vi "Obtain Channel DBL.vi"(8 "error in (no error)":errorcluster, 10 "Name":string, 11 "VolatusAPI in":refnum<class "VolatusAPI.lvclass">) -> (0 "error out":errorcluster, 2 "Channel DBL":refnum<class "Channel DBL.lvclass">, 3 "VolatusAPI out":refnum<class "VolatusAPI.lvclass">)   [LabVIEW 2020, in "Volatus.lvlib" / "VolatusAPI.lvclass"]
uses:
  VolatusAPI.lvclass
  VolatusAPI.lvclass/VolatusAPI.ctl
  lv-vecto/Vecto/Group DBL/Group DBL.lvclass
  C:/dev/lv20CE/relink/lv-vecto/Vecto/Group/Group.lvclass
  C:/dev/lv20CE/relink/lv-vecto/Vecto/Group DBL/Group DBL.lvclass
  lv-vecto/Vecto/Channel DBL/Channel DBL.lvclass
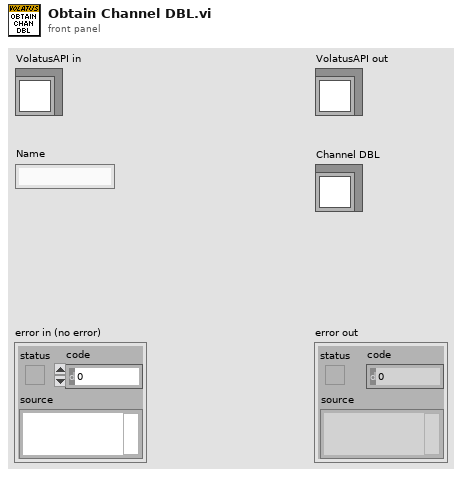
[diagram p1: front panel]
types:
  T1 = typedef "VectoConfig.lvlib/Channel Info.ctl" = cluster{"Name":string, "Group":string, "Owning Node":string, "Owning Task":string, "Resource":string}
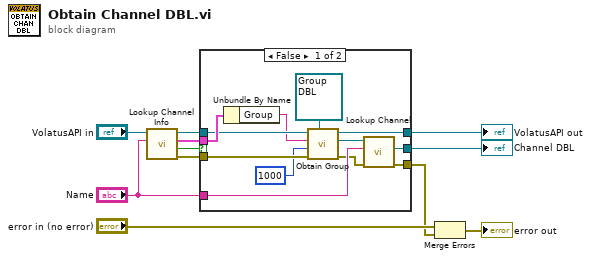
[diagram p0: block diagram]
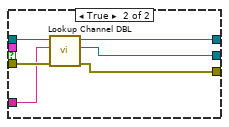
[diagram p2: hidden frame]
diagram:
  n1 = call "Lookup Channel Info.vi"("Channel Name"="Name", "VolatusAPI in"="VolatusAPI in") -> ("error out"=w5:errorcluster, "Local"=w7:bool, "Channel Info"=w8:T1, "VolatusAPI out"=w9:refnum<class "VolatusAPI.lvclass">)  [unwired: 5 in, 1 out]
  n2 = case shown="False" w7 {
    tunnel: w9 -> [w22 w28]
    tunnel: w8 -> [w23 _]
    tunnel: "Name" -> [w16 w27]
    tunnel: w5 -> [w19 w29]
    tunnel: [w12 w26] -> w4
    tunnel: [w13 w25] -> w3
    tunnel: [w14 w24] -> w1
    frame False {
      n3 = Unbundle By Name(w23) -> ("Group"=w20:string)
      n4 = call "Obtain Group.vi"("Group Type (Abstract)"=refnum<class "Group DBL.lvclass"> refnum ("Vecto.lvlib:Group DBL.lvclass"), "error in (no error)"=w19, "Timeout ms (5000)"=u32 1000, "Group Name"=w20, "VolatusAPI in"=w22) -> ("error out"=w15:errorcluster, "Group"=w17:refnum<class "Group DBL.lvclass">, "VolatusAPI out"=w12:refnum<class "VolatusAPI.lvclass">)  [unwired: 4 in]
      n5 = call "Lookup Channel.vi"("error in (no error)"=w15, "Channel Name"=w16, "Group in"=w17) -> ("error out"=w14:errorcluster, "Channel"=w13:refnum<class "Channel DBL.lvclass">)  [unwired: 6 in, 1 out]
    }
    frame True {
      n6 = call "Lookup Channel DBL.vi"("error in (no error)"=w29, "Name"=w27, "VolatusAPI in"=w28) -> ("error out"=w24:errorcluster, "Channel DBL"=w25:refnum<class "Channel DBL.lvclass">, "VolatusAPI out"=w26:refnum<class "VolatusAPI.lvclass">)  [unwired: 6 in]
    }
  }
  "VolatusAPI out" <- w4
  "Channel DBL" <- w3
  n7 = Merge Errors("error in (no error)", w1) -> (→"error out":errorcluster)
